vi "PostCopyScripting.vi"(10 "metadataobj":refnum<class "MetaDataObj.lvclass">, 11 "user project":refnum<vi>) -> ()   [LabVIEW 2013, in "DecideModuleFeatures.lvclass"]
uses:
  DecideModuleFeatures.lvclass
  <resource>/dialog/NewProjectWizard/MetaDataObj/MetaDataObj.lvclass
  DecideModuleFeatures.lvclass/DecideModuleFeatures.ctl
  Read component name.vi
  <vilib>/Utility/EditLVLibs/Edit LVLibs.lvlib
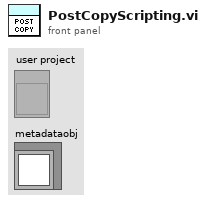
[diagram p1: front panel]
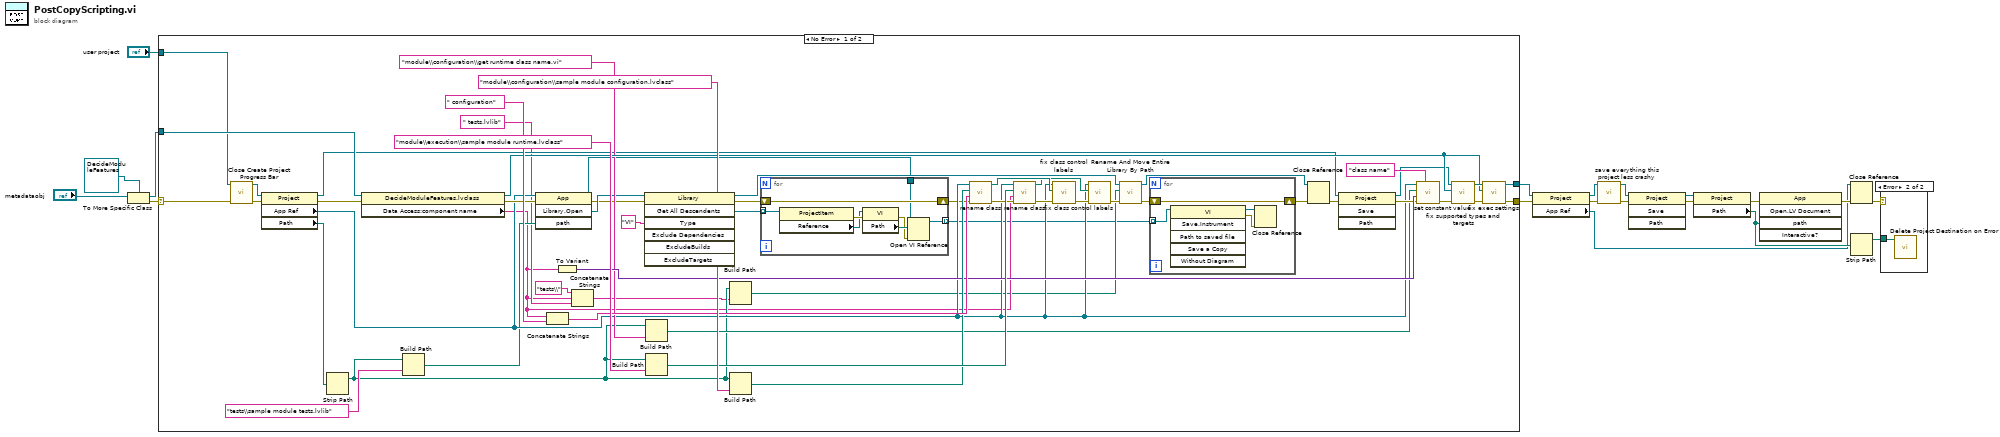
[diagram p0: block diagram]
diagram:
  n1 = To More Specific Class(target class=refnum<class "DecideModuleFeatures.lvclass"> refnum ("DecideProjectFeatures.lvclass"), reference="metadataobj") -> (specific class reference=w10:refnum<class "DecideModuleFeatures.lvclass">, error out=w17:errorcluster)  [unwired: 1 in]
  n2 = case shown="No Error" w17 {
    selector: w17 -> [w48 w87]
    tunnel: [w62 w88] -> w7
    tunnel: "user project" -> [w47 w88]
    tunnel: [w61 w87] -> w6
    tunnel: w10 -> [w70 _]
    frame No Error {
      n3 = call <resource>:"Close Create Project Progress Bar.vi"("error in (no error)"=w48, "Project"=w47) -> ("error out"=w45:errorcluster, "dup Project"=w46:refnum<vi>)  [unwired: 8 in]
      n4 = property class="Project"(reference=w46, error in=w45) -> (reference out=w54:refnum<vi>, error out=w74:errorcluster, "App Ref"=w41:refnum<vi>, "Path"=w73:path)
      n5 = Strip Path(path=w73) -> (stripped path=w39:path)  [unwired: 1 out]
      n6 = property class="DecideModuleFeatures.lvclass"(reference=w70, error in=w74) -> (reference out=w59:refnum<class "DecideModuleFeatures.lvclass">, error out=w64:errorcluster, "Data Access:component name"=w35:string)
      n7 = Build Path(base path=w39, name or relative path="tests\\sample module tests.lvlib") -> (appended path=w40:path)
      n8 = invoke class="App" method="Library.Open"(reference=w41, error in=w64, "path"=w40) -> (reference out=w20:refnum<vi>, error out=w26:errorcluster, "Open Library"=w28:refnum<vi>)  [unwired: 1 in, 1 out]
      n9 = Concatenate Strings(w35, " configuration" ("string")) -> (w66:string)
      n10 = To Variant(anything=w35) -> (Variant=w58:variant)
      n11 = Concatenate Strings("tests\\" ("name or relative path"), w35, " tests.lvlib" ("name or relative path")) -> (w36:string)
      n12 = invoke class="Library" method="Get All Descendents"(reference=w28, error in=w26, "Type"="VI") -> (reference out=w27:refnum<vi>, error out=w22:errorcluster, "All Descendents"=w29:refnum<vi>[])  [unwired: 4 in, 4 out]
      n13 = Build Path(base path=w39, name or relative path="module\\configuration\\get runtime class name.vi") -> (appended path=w43:path)
      n14 = Build Path(base path=w39, name or relative path="module\\execution\\sample module runtime.lvclass") -> (appended path=w69:path)
      n15 = Build Path(base path=w39, name or relative path=w36) -> (appended path=w31:path)
      n16 = Build Path(base path=w39, name or relative path="module\\configuration\\sample module configuration.lvclass") -> (appended path=w65:path)
      n17 = for {
        tunnel: w29 -> [w86] mode=indexing
        tunnel: [w81] -> w23 mode=indexing
        shift-right: [w80] -> w21
        shift-left: w22 -> [w80]
        tunnel: w20 -> [w79]
        n18 = property class="ProjectItem"(reference=w86) -> (error out=w85:errorcluster, "Reference"=w84:refnum<vi>)  [unwired: 1 in, 1 out]
        n19 = property class="VI"(reference=w84, error in=w85) -> (error out=w82:errorcluster, "Path"=w83:path)  [unwired: 1 out]
        n20 = Open VI Reference(application reference (local)=w79, vi path=w83, error in (no error)=w82) -> (vi reference=w81:refnum<vi>)  [unwired: 3 in, 1 out]
      }
      n21 = call "rename class.vi"("error in"=w21, "new name"=w66, "class path"=w65, "application in"=w41) -> ("error out"=w67:errorcluster, "new library path"=w52:path)  [unwired: 6 in]
      n22 = call "rename class.vi"("error in"=w67, "new name"=w35, "class path"=w69, "application in"=w41) -> ("error out"=w51:errorcluster, "new library path"=w49:path)  [unwired: 6 in]
      n23 = call "fix class control labels.vi"("error in"=w51, "class to load"=w52, "application in"=w41) -> ("error out"=w50:errorcluster)  [unwired: 8 in]
      n24 = call "fix class control labels.vi"("error in"=w50, "class to load"=w49, "application in"=w41) -> ("error out"=w34:errorcluster)  [unwired: 8 in]
      n25 = call <vilib>:"Rename And Move Entire Library By Path.vi"("error in (no error)"=w34, "New library path"=w31, "Library ref in"=w27) -> ("error out"=w25:errorcluster, "Library ref out"=w32:refnum<vi>)  [unwired: 7 in]
      n26 = for {
        tunnel: w23 -> [w78] mode=indexing
        shift-right: [w75] -> w24
        shift-left: w25 -> [w75]
        n27 = invoke class="VI" method="Save.Instrument"(reference=w78) -> (reference out=w76:refnum<vi>, error out=w77:errorcluster)  [unwired: 5 in, 4 out]
        n28 = Close Reference(reference=w76, error in (no error)=w77) -> ()  [unwired: 1 out]
      }
      n29 = Close Reference(reference=w32, error in (no error)=w24) -> (error out=w33:errorcluster)
      n30 = invoke class="Project" method="Save"(reference=w54, error in=w33) -> (reference out=w53:refnum<vi>, error out=w55:errorcluster)  [unwired: 2 in, 2 out]
      n31 = call "set constant value.vi"("control name"="class name", "error in"=w55, "data to set"=w58, "vi path"=w43, "application in"=w41) -> ("error out"=w44:errorcluster)  [unwired: 6 in]
      n32 = call "fix supported types and targets.vi"("error in"=w44, "decideprojectfeatures in"=w59, "user project in"=w53) -> ("error out"=w60:errorcluster, "user project out"=w63:refnum<vi>)  [unwired: 7 in]
      n33 = call "fix exec settings.vi"("error in"=w60, "decideprojectfeatures in"=w59, "user project in"=w63) -> ("error out"=w61:errorcluster, "user project out"=w62:refnum<vi>)  [unwired: 7 in]
    }
    frame Error {
    }
  }
  n34 = property class="Project"(reference=w7, error in=w6) -> (reference out=w4:refnum<vi>, error out=w5:errorcluster, "App Ref"=w3:refnum<vi>)
  n35 = call "save everything this project less crashy.vi"("error in"=w5, "project in"=w4) -> ("error out"=w9:errorcluster, "project out"=w8:refnum<vi>)  [unwired: 8 in]
  n36 = invoke class="Project" method="Save"(reference=w8, error in=w9) -> (reference out=w13:refnum<vi>, error out=w14:errorcluster)  [unwired: 2 in, 2 out]
  n37 = property class="Project"(reference=w13, error in=w14) -> (error out=w16:errorcluster, "Path"=w11:path)  [unwired: 1 out]
  n38 = invoke class="App" method="Open.LV Document"(error in=w16, "path"=w11) -> (error out=w15:errorcluster)  [unwired: 3 in, 4 out]
  n39 = Close Reference(reference=w3, error in (no error)=w15) -> (error out=w2:errorcluster)
  n40 = Strip Path(path=w11) -> (stripped path=w1:path)  [unwired: 1 out]
  n41 = case shown="Error" w2 {
    tunnel: w1 -> [_ w89]
    frame No Error {
    }
    frame Error {
      n42 = call <resource>:"Delete Project Destination on Error.vi"("Project Destination Root"=w89) -> ()  [unwired: 11 in]
    }
  }
